vi "Write Resource Name.vi"(8 "error in (no error)":errorcluster, 10 "Resource Name":refnum<visa-resource-name>, 11 "ACM4509 in":refnum<class "Cal Standard.lvclass">) -> (0 "error out":errorcluster, 3 "ACM4509 out":refnum<class "Cal Standard.lvclass">)   [LabVIEW 2023, in "ACM 4509 Cal Standard.lvlib" / "Cal Standard.lvclass"]
uses:
  Cal Standard.lvclass
  Cal Standard.lvclass/Cal Standard.ctl
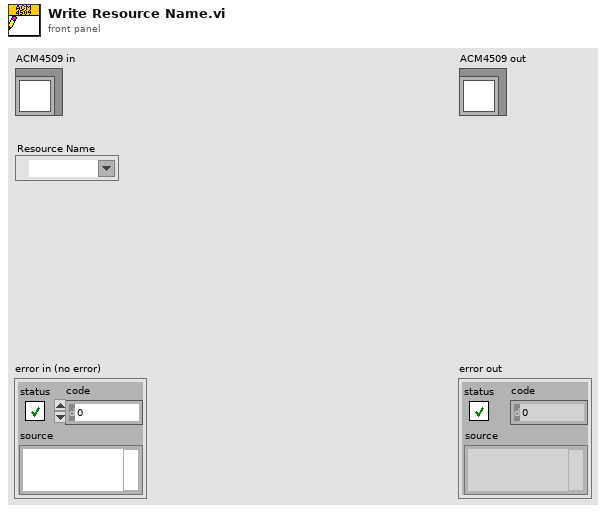
[diagram p1: front panel]
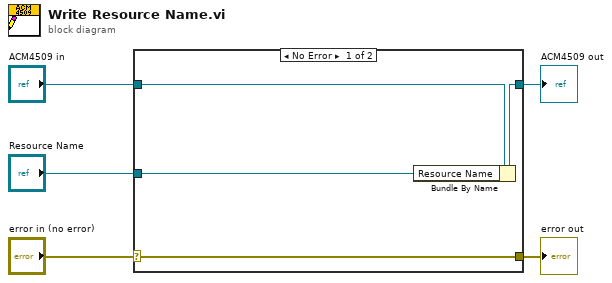
[diagram p0: block diagram]
diagram:
  n1 = case shown="No Error" "error in (no error)" {
    selector: "error in (no error)" -> [w9 w10]
    tunnel: [w9 w10] -> w4
    tunnel: [w7 w11] -> w2
    tunnel: "ACM4509 in" -> [w8 w11]
    tunnel: "Resource Name" -> [w6 _]
    frame No Error {
      n2 = Bundle By Name(cluster=w8, "Resource Name"=w6) -> (w7:refnum<class "Cal Standard.lvclass">)
    }
    frame Error {
    }
  }
  "error out" <- w4
  "ACM4509 out" <- w2
